vi "DV - Read desired velocity.vi"(1 "Address / Port":i16=1 min=1 max=31 step=1, 2 "error in":errorcluster, 3 "Axis":i8=1 min=1 max=6 step=1) -> (0 "error out":errorcluster)   [LabVIEW 2014]
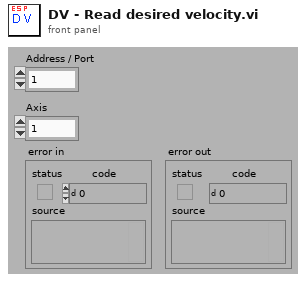
[diagram p1: front panel]
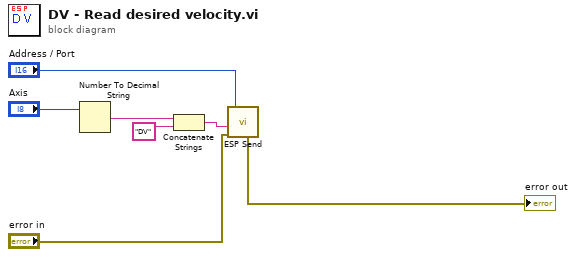
[diagram p0: block diagram]
diagram:
  n1 = Number To Decimal String(number="Axis") -> (decimal integer string=w6:string)  [unwired: 1 in]
  n2 = Concatenate Strings(w6, "DV" ("Substring")) -> (w4:string)
  n3 = call "ESP Send.vi"("Address / Port"="Address / Port", "Command String"=w4, "error in"="error in") -> ("error out"=→"error out":errorcluster)  [unwired: 5 in]
